vi "Target.vi"() -> ()   [LabVIEW 2017]
uses:
  shared/Kobuki Sensor Display.ctl
  controls/StatesEnum.ctl
  <vilib>/Platform/TimedLoop/XDataNode/timing_clust.ctl
  <vilib>/Platform/TimedLoop/XDataNode/nitl_modes.ctl
  <vilib>/Platform/TimedLoop/XDataNode/wakeup.ctl
  <vilib>/myRIO/Instrument Drivers/Onboard IO/UART/typedef/VISA Configuration.ctl
  shared/Sensors.ctl
  shared/Accelerometer.ctl
  Kobuki/KobukiSensors.ctl
  Kobuki/Kobuki Bumps and WheelDrops.ctl
  Kobuki/Kobuki Buttons.ctl
  <vilib>/myRIO/Common/Instrument Driver Framework/myRIO v1.0/UART/vis/myRIO v1.0 Close UART.vi
  <vilib>/myRIO/Common/Instrument Driver Framework/myRIO v1.0/myRIO v1.1 Open.vi
  <vilib>/Instr/_visa.llb/VISA Configure Serial Port (Instr).vi
  <vilib>/myRIO/Common/Instrument Driver Framework/Utilities/vis/FPGA Ref Manager.vi
  <vilib>/myRIO/Common/Instrument Driver Framework/myRIO v1.0/myRIO v1.0 Reset FPGA.vi
  <vilib>/myRIO/Common/Instrument Driver Framework/myRIO v1.0/IRQ/vis/myRIO v1.0 IRQ Info FGV.vi
  <vilib>/myRIO/Common/Instrument Driver Framework/myRIO v1.0/IRQ/vis/myRIO v1.0 Timer IRQ Info FGV.vi
  <vilib>/myRIO/Common/Instrument Driver Framework/myRIO v1.0/IRQ/vis/myRIO v1.0 ISR Agent.vi
  <vilib>/Platform/TimedLoop/XDataNode/XDataNode.xnode
  <vilib>/myRIO/Express VI/Onboard IO/UART/UART Express VI.xnode
  <vilib>/myRIO/Instrument Drivers/Utilities/Utilities.lvlib
  <vilib>/Platform/TimedLoop/XDataNode/XDNodeRunTimeDep.lvlib
  <vilib>/myRIO/Instrument Drivers/Onboard IO/UART/UART.lvlib
panel:
  in  "Pause":bool
  in  "Tab Control":T1(tab)
  out "Kobuki Sensors (graphical)":T2 {"Right Wheel (mm/s)" scale=-500.0..500.0; "Left Wheel (mm/s)" scale=-500.0..500.0}
  out "Charge Status":i8(ring) items=["DISCHARGING"=0, "DOCKING_CHARGED"=2, "DOCKING_CHARGING"=6, "ADAPTER_CHARGED"=18, "ADAPTER_CHARGING"=22]
  out "Kobuki Battery Voltage":dbl(knob)=12000.0 scale=12.0..16.4 scale format="%#.1f"
  out "CurrentState":T4
  out "Loop Duration":i64
  out "error out":errorcluster
  in  "stop":bool
  out "Target Running":bool
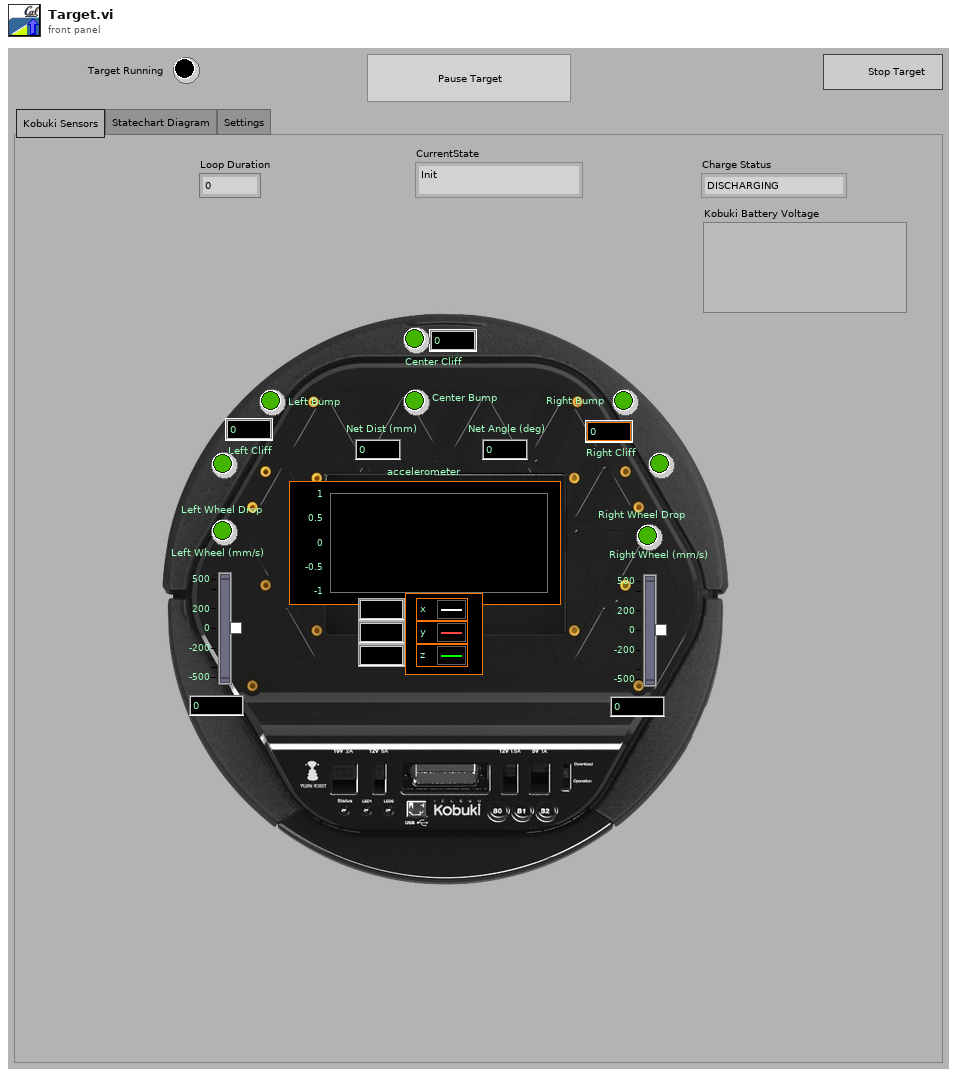
[diagram p1: front panel]
types:
  T1 = enum32{"Kobuki Sensors", "Statechart Diagram", "Settings"}
  T2 = typedef "Kobuki Sensor Display.ctl" = cluster{"Center Bump":bool, "Left Wheel Drop":bool, "Right Wheel Drop":bool, "Left Bump":bool, "Right Bump":bool, "Left Cliff":bool, "Center Cliff":bool, "Right Cliff":bool, "Net Dist (mm)":i32, "Net Angle (deg)":i32, "Left Cliff":u16, "Center Cliff":u16, "Right Cliff":u16, "  Left Wheel (mm/s)":i16, "Right Wheel (mm/s)":i16, "accelerometer":T3}
  T3 = typedef "Accelerometer.ctl" = cluster{"x axis (g)":dbl, "y axis (g)":dbl, "z axis (g)":dbl}
  T4 = typedef "StatesEnum.ctl" = enum16{"Init", "Center Cliff\n", "Pause", "Drive", "L.Cliff", "R.Cliff", "Shut"}
  T5 = typedef "XDNodeRunTimeDep.lvlib/timing_clust.ctl" = cluster{"Expected End [f-1]":u64, "Actual End [f-1]":u64, "Finished Late? [f-1]":bool, "Expected End [i-1]":u64, "Actual End [i-1]":u64, "Finished Late? [i-1]":bool, "Expected Start [i]":u64, "Actual Start [i]":u64, "Expected Start [f]":u64, "Actual Start [f]":u64, "Source Name":string, "Structure Name":string, "Period":i64, "Deadline":i64, "Offset":i64, "Start":i64, "Priority":i32, "Timeout":i32, "Mode":T6, "Wakeup Reason":T7, "Error":errorcluster, "Source Type":string, "Secondary Source Type":string, "Global End Time":u64, "Global Start Time":u64, "Frame Duration":u64, "Iteration Duration":u64, "Assigned CPU":i32, "I/O Scan Engine Mode":u32}
  T6 = typedef "XDNodeRunTimeDep.lvlib/nitl_modes.ctl" = enum32{"No Change", "Process missed periods, maintain original phase", "Discard missed periods, maintain original phase", "Process missed periods, ignore original phase", "Discard missed periods, ignore original phase"}
  T7 = typedef "XDNodeRunTimeDep.lvlib/wakeup.ctl" = enum32{"Normal", "Aborted", "Asynchronous wakeup", "Timing source error", "Timed loop error", "Timeout"}
  T8 = typedef "Sensors.ctl" = cluster{"net distance (mm)":i32, "net angle (deg)":i32, "accelerometer":T3, "Is Simulator?":bool, "Kobuki Sensors":T9, "Requested Left Wheel Velocity(mm/s)":i32, "Requested Right Wheel Velocity(mm/s)":i32}
  T9 = typedef "KobukiSensors.ctl" = cluster{"Bumps + Wheel Drops":T10, "Cliff Left":bool, "Cliff Center":bool, "Cliff Right":bool, "Cliff Left Signal":u16, "Cliff Center Signal":u16, "Cliff Right Signal":u16, "Buttons":T11, "Left Wheel Encoder (ticks)":u16, "Right Wheel Encoder (ticks) ":u16, "Left  Wheel PWM":i8, "Right Wheel PWM":i8, "Left Wheel OverCurrent":bool, "Right Wheel OverCurrent ":bool, "Right Wheel Current (x10mA)":i16, "Left  Wheel Current  (x10mA)":i16, "TimeStamp":u16, "Battery Voltage":dbl, "Angle( of 100deg)":i16, "Angle Rate( of 100 deg/sec)":i16, "Charger Source ":i8}
  T10 = typedef "Kobuki Bumps and WheelDrops.ctl" = cluster{"Wheeldrop Left":bool, "Wheeldrop Right":bool, "Bump Left":bool, "Bump Center":bool, "Bump Right":bool}
  T11 = typedef "Kobuki Buttons.ctl" = cluster{"B0":bool, "B1":bool, "B2":bool}
  T12 = typedef "Outputs.ctl" = cluster{"Left Wheel Speed (mm/s)":i16, "Right Wheel Speed (mm/s)":i16}
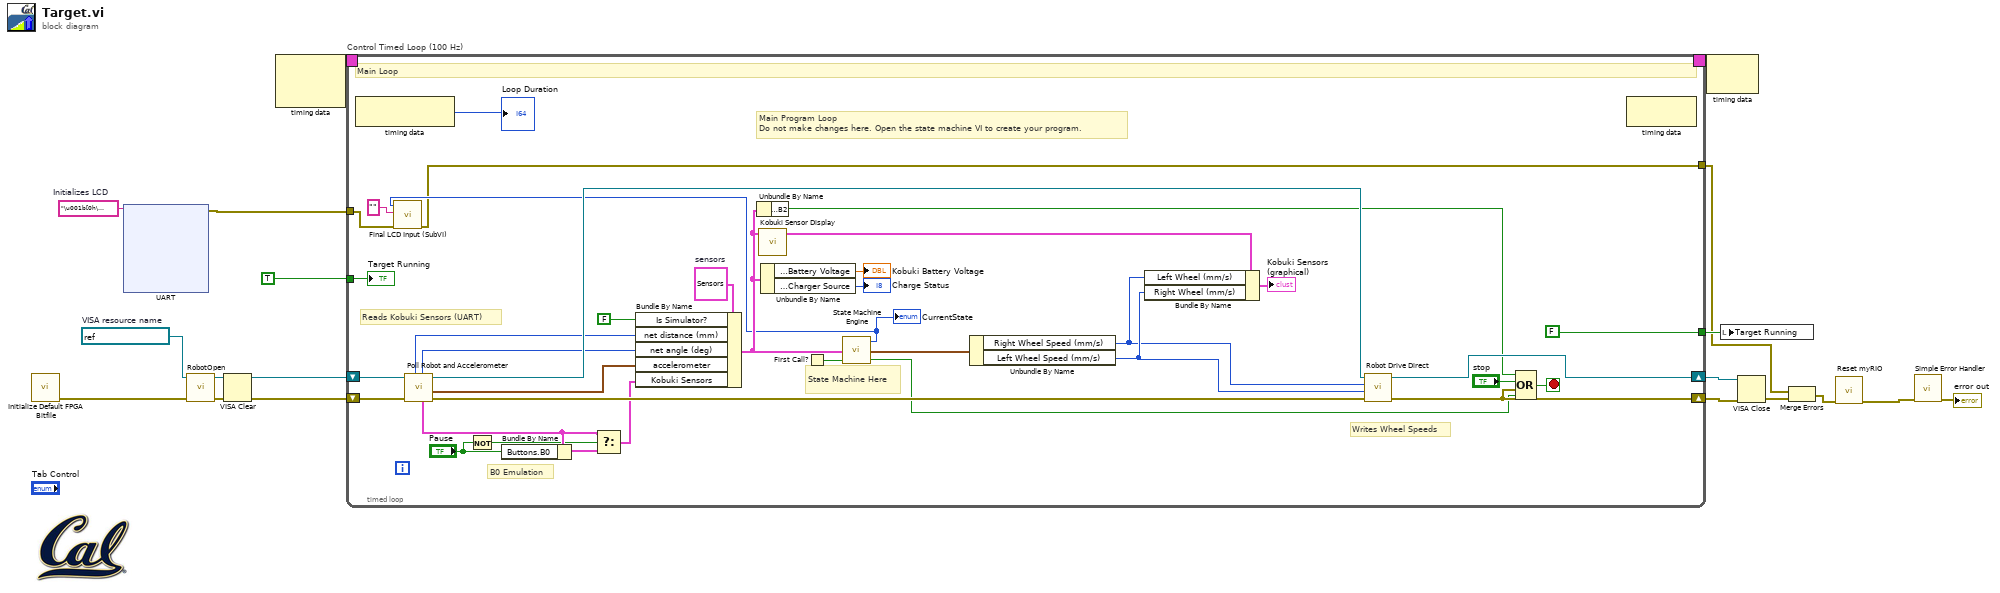
[diagram p0: block diagram]
diagram:
  w4 = "\u001b[0h\u001b[j"  # Initializes LCD
  w16 = refnum<visa-resource-name> "ASRL3::INSTR"  # VISA resource name
  n1 = call <vilib>:"Initialize Default FPGA Bitfile.vi"() -> ("error out"=w14:errorcluster)  [unwired: 11 in]
  n2 = xnode "UART"("Characters to Write"=w4) -> ("error out"=w5:errorcluster)  [unwired: 1 in, 1 out]
  n3 = call "RobotOpen.vi"("error in (no error)"=w14, "Robot Communication port name"=w16) -> ("error out"=w12:errorcluster, "Robot Communication port name out"=w19:refnum<visa-resource-name>)  [unwired: 8 in]
  n4 = VISA Clear(VISA resource name=w19, error in (no error)=w12) -> (VISA resource name out=w10:refnum<visa-resource-name>, error out=w11:errorcluster)
  n5 = node-c288() -> (w7:T5)  [unwired: 2 in]
  n6 = timed-loop "Control Timed Loop (100 Hz)" {
    shift-right: [w55] -> w8
    shift-left: w10 -> [w52]
    shift-right: [w40] -> w9
    shift-left: w11 -> [w51]
    tunnel: TRUE ("stop") -> [w46]
    tunnel: [FALSE ("stop")] -> w17
    timing: w7 -> [_]
    timing-out: [_] -> w6
    tunnel: w5 -> [w23]
    tunnel: [w20] -> w2
    stop <- w54 stop-if-true
    w41 = T8 {"net distance (mm)"=0, "net angle (deg)"=0, "accelerometer"={"x axis (g)"=0.0, "y axis (g)"=0.0, "z axis (g)"=0.0}, "Is Simulator?"=FALSE, "Kobuki Sensors"={"Bumps + Wheel Drops"={"Wheeldrop Left"=FALSE, "Wheeldrop Right"=FALSE, "Bump Left"=FALSE, "Bump Center"=FALSE, "Bump Right"=FALSE}, "Cliff Left"=FALSE, "Cliff Center"=FALSE, "Cliff Right"=FALSE, "Cliff Left Signal"=0, "Cliff Center Signal"=0, "Cliff Right Signal"=0, "Buttons"={"B0"=FALSE, "B1"=FALSE, "B2"=FALSE}, "Left Wheel Encoder (ticks)"=0, "Right Wheel Encoder (ticks) "=0, "Left  Wheel PWM"=0, "Right Wheel PWM"=0, "Left Wheel OverCurrent"=FALSE, "Right Wheel OverCurrent "=FALSE, "Right Wheel Current (x10mA)"=0, "Left  Wheel Current  (x10mA)"=0, "TimeStamp"=0, "Battery Voltage"=0.0, "Angle( of 100deg)"=0, "Angle Rate( of 100 deg/sec)"=0, "Charger Source "=0}, "Requested Left Wheel Velocity(mm/s)"=0, "Requested Right Wheel Velocity(mm/s)"=0}  # sensors
    # "B0 Emulation"
    # "Main Program Loop\nDo not make changes here. Open the state machine VI to create your program."
    # "Writes Wheel Speeds"
    # "Reads Kobuki Sensors (UART)"
    # "State Machine Here"
    # "Main Loop"
    n7 = node-c288() -> (→"Loop Duration":i64)  [unwired: 1 in]
    n8 = call "Poll Robot and Accelerometer.vi"("error in"=w51, "UART in"=w52) -> ("error out"=w50:errorcluster, "Acceleration (g)"=w43:T3, "UART out"=w49:refnum<visa-resource-name>, "Kobuki Sensors  out"=w27:T9, "net angle (deg)"=w47:i32, "net distance (mm)"=w48:i32)  [unwired: 4 in]
    n9 = Not(x="Pause") -> (.not. x?=w24:bool)
    n10 = Bundle By Name(cluster=w27, "Buttons.B0"="Pause") -> (w28:T9)
    n11 = Select(t=w27, s=w24, f=w28) -> (s? t:f=w26:T9)
    n12 = Bundle By Name(cluster=w41, "Is Simulator?"=FALSE, "net distance (mm)"=w48, "net angle (deg)"=w47, "accelerometer"=w43, "Kobuki Sensors"=w26) -> (w33:T8)
    n13 = Unbundle By Name(w33) -> ("Kobuki Sensors.Buttons.B2"=w44:bool)
    n14 = call "Kobuki Sensor Display.vi"("sensors"=w33) -> ("Kobuki Sensors Display"=w30:T2)  [unwired: 4 in]
    n15 = Unbundle By Name(w33) -> ("Kobuki Sensors.Battery Voltage"=→"Kobuki Battery Voltage":dbl, "Kobuki Sensors.Charger Source"=→"Charge Status":i8)
    n16 = First Call?() -> (First Call?: T/F=w35:bool)
    n17 = call "State Machine Engine.vi"("Init?"=w35, "Inputs"=w33) -> ("Terminated?"=w34:bool, "Outputs"=w38:T12, "state out"=w21:T4)  [unwired: 1 in]
    "CurrentState" <- w21
    n18 = call "Final LCD Input (SubVI).vi"("error in (no error)"=w23, "String Input"="", "state input"=w21) -> ("error out"=w20:errorcluster)  [unwired: 8 in]
    n19 = Unbundle By Name(w38) -> ("Right Wheel Speed (mm/s)"=w31:i16, "Left Wheel Speed (mm/s)"=w32:i16)
    n20 = Bundle By Name(cluster=w30, "Left Wheel (mm/s)"=w31, "Right Wheel (mm/s)"=w32) -> (→"Kobuki Sensors (graphical)":T2)
    n21 = call "Robot Drive Direct.vi"("error in"=w50, "Left Wheel Velocity (mm/s)"=w32, "Right Wheel Velocity (mm/s)"=w31, "UART port in"=w49) -> ("error out"=w40:errorcluster, "UART port out"=w55:refnum<visa-resource-name>)  [unwired: 6 in]
    n22 = Compound Arithmetic op=OR(w44, "stop", w40, w34) -> (w54:bool)
    n23 = node-c288() -> ()  [unwired: 1 in, 1 out]
    "Target Running" <- w46
  }
  n24 = node-c288(w6) -> ()  [unwired: 1 out]
  n25 = local write "Target Running"(w17) -> ()
  n26 = VISA Close(VISA resource name=w8, error in (no error)=w9) -> (error out=w3:errorcluster)
  n27 = Merge Errors(w2, w3) -> (w1:errorcluster)
  n28 = call <vilib>:"Reset myRIO.vi"("error in (no error)"=w1) -> ("error out"=w15:errorcluster)  [unwired: 10 in]
  n29 = call <vilib>:"Simple Error Handler.vi"("error in (no error)"=w15) -> ("error out"=→"error out":errorcluster)  [unwired: 4 in, 4 out]
